vi "circular_shooter_calc.vi"(9 "Shooting Speed":dbl=3.0, 10 "Shooter_Inputs":T1, 11 "Circular Shooter Commands":T3) -> (3 "Shooter_Outputs":T2)   [LabVIEW 2012]
uses:
  circular_shooter_commands.ctl
  Shooter_Outputs.ctl
  Shooter_inputs.ctl
panel:
  in  "Dejam Speed":dbl=-3.0
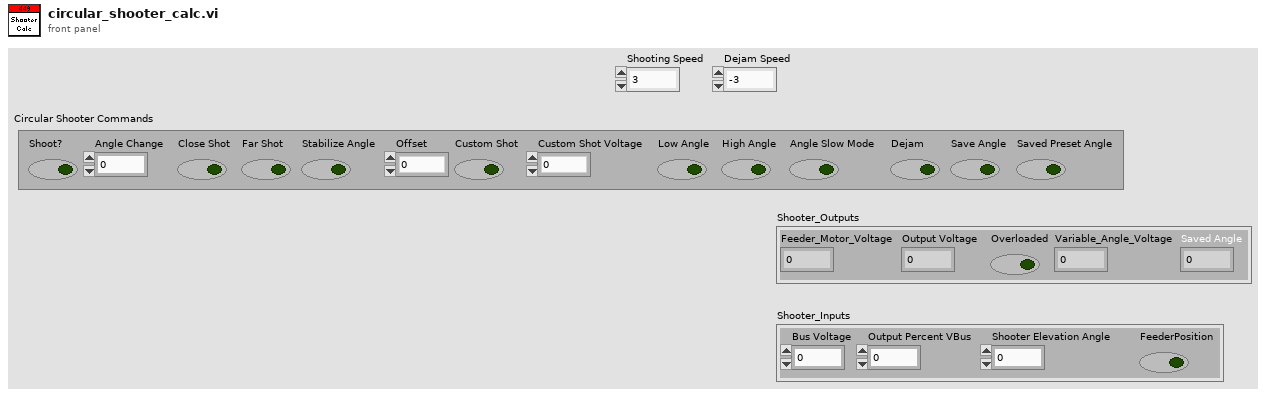
[diagram p1: front panel]
types:
  T1 = typedef "Shooter_inputs.ctl" = cluster{"Bus Voltage":dbl, "Output Percent VBus":dbl, "Shooter Elevation Angle":dbl, "FeederPosition":bool}
  T2 = typedef "Shooter_Outputs.ctl" = cluster{"Feeder_Motor_Voltage":dbl, "Output Voltage":dbl, "Overloaded":bool, "Variable_Angle_Voltage":dbl, "Saved Angle":dbl}
  T3 = typedef "circular_shooter_commands.ctl" = cluster{"Shoot?":bool, "Angle Change":dbl, "Close Shot":bool, "Far Shot":bool, "Stabilize Angle ":bool, "Offset":dbl, "Custom Shot":bool, "Custom Shot Voltage":dbl, "Low Angle":bool, "High Angle":bool, "Angle Slow Mode":bool, "Dejam":bool, "Save Angle":bool, "Saved Preset Angle":bool}
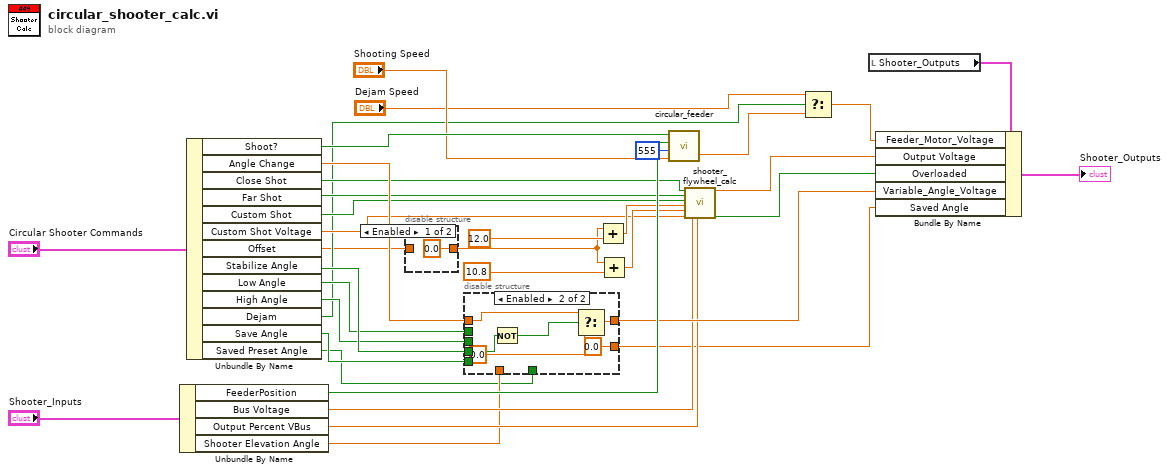
[diagram p0: block diagram]
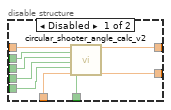
[diagram p3: hidden frame]
diagram:
  n1 = Unbundle By Name("Shooter_Inputs") -> ("FeederPosition"=w30:bool, "Bus Voltage"=w23:dbl, "Output Percent VBus"=w24:dbl, "Shooter Elevation Angle"=w13:dbl)
  n2 = Unbundle By Name("Circular Shooter Commands") -> ("Shoot?"=w12:bool, "Angle Change"=w34:dbl, "Close Shot"=w20:bool, "Far Shot"=w19:bool, "Custom Shot"=w16:bool, "Custom Shot Voltage"=w17:dbl, "Offset"=w5:dbl, "Stabilize Angle"=w18:bool, "Low Angle"=w15:bool, "High Angle"=w14:bool, "Dejam"=w7:bool, "Save Angle"=w3:bool, "Saved Preset Angle"=w2:bool)
  n3 = disable-structure shown="Enabled" {
    disable-tunnel: w5 -> [_ w37]
    disable-tunnel: [0.0 ("Offset") w37] -> w4
    frame Enabled {
    }
    frame Disabled {
    }
  }
  n4 = disable-structure shown="Enabled" {
    disable-tunnel: w34 -> [w45 w52]
    disable-tunnel: [w46 w51] -> w29
    disable-tunnel: w18 -> [w44 w50]
    disable-tunnel: w15 -> [w43 _]
    disable-tunnel: w14 -> [w42 _]
    disable-tunnel: w13 -> [w41 _]
    disable-tunnel: w3 -> [w40 _]
    disable-tunnel: w2 -> [w39 _]
    disable-tunnel: [w38 0.0 ("Saved Angle")] -> w1
    frame Disabled {
      n5 = call "circular_shooter_angle_calc_v2.vi"("Driver Input"=w45, "Low Angle"=w43, "High Angle"=w42, "Stabalize Angle"=w44, "Save Angle"=w40, "Current Angle"=w41, "Saved Angle Preset"=w39) -> ("Motor Voltage Out"=w46:dbl, "Saved Angle"=w38:dbl)  [unwired: 11 in]
    }
    frame Enabled {
      n6 = Not(x=w50) -> (.not. x?=w49:bool)
      n7 = Select(t=w52, s=w49, f=0.0) -> (s? t:f=w51:dbl)
    }
  }
  n8 = Add(x=w4, y=12.0 ("Close Voltage")) -> (x+y=w22:dbl)
  n9 = Add(x=w4, y=10.8 ("Far Voltage")) -> (x+y=w21:dbl)
  n10 = call "circular_feeder.vi"("Shoot"=w12, "Limit Switch"=w30, "Dt"=u32 555, "Spinning Speed"="Shooting Speed") -> ("Motor Voltage"=w10:dbl)  [unwired: 1 in, 1 out]
  n11 = call "shooter_flywheel_calc.vi"("Close Shot"=w20, "Far Shot"=w19, "Custom Shot"=w16, "Close Voltage"=w22, "Far Voltage"=w21, "Custom Shot Voltage"=w17, "Bus Voltage"=w23, "Output Percent VBus"=w24) -> ("Voltage Output"=w27:dbl, "Overloaded"=w28:bool)  [unwired: 10 in]
  n12 = Select(t="Dejam Speed", s=w7, f=w10) -> (s? t:f=w9:dbl)
  n13 = local read "Shooter_Outputs"() -> (w32:T2)
  n14 = Bundle By Name(cluster=w32, "Feeder_Motor_Voltage"=w9, "Output Voltage"=w27, "Overloaded"=w28, "Variable_Angle_Voltage"=w29, "Saved Angle"=w1) -> (→"Shooter_Outputs":T2)
